vi "BindCluster.vi"(8 "error in (no error)":errorcluster, 9 "Controls[]":refnum<vi>[](array[refnum]), 10 "Cols":T2[](array[typedef])=[{"Include"=TRUE, "Name"="Position", "SQLite3 type"=enum."SQLITE_FLOAT"}, {"Include"=TRUE, "Name"="Event Type", "SQLite3 type"=enum."SQLITE_INTEGER"}, {"Include"=TRUE, "Name"="Area", "SQLite3 type"=enum."SQLITE_INTEGER"}, {"Include"=TRUE, "Name"="Channels", "SQLite3 type"=enum."SQLITE_INTEGER"}, {"Include"=TRUE, "Name"="Start position", "SQLite3 type"=enum."SQLITE_INTEGER"}, {"Include"=TRUE, "Name"="End  position", "SQLite3 type"=enum."SQLITE_INTEGER"}, {"Include"=TRUE, "Name"="Name", "SQLite3 type"=enum."SQLITE3_TEXT"}, {"Include"=TRUE, "Name"="Offset", "SQLite3 type"=enum."SQLITE_INTEGER"}, {"Include"=TRUE, "Name"="Length", "SQLite3 type"=enum."SQLITE_INTEGER"}, {"Include"=TRUE, "Name"="Action marker", "SQLite3 type"=enum."SQLITE3_TEXT"}, {"Include"=TRUE, "Name"="Event", "SQLite3 type"=enum."SQLITE_INTEGER"}, {"Include"=TRUE, "Name"="# Defects", "SQLite3 type"=enum."SQLITE_INTEGER"}, {"Include"=TRUE, "Name"="jpg Image", "SQLite3 type"=enum."SQLITE3_TEXT"}, {"Include"=TRUE, "Name"="chan maxs", "SQLite3 type"=enum."SQLITE_INTEGER"}, {"Include"=TRUE, "Name"="chan mins", "SQLite3 type"=enum."SQLITE_INTEGER"}, {"Include"=TRUE, "Name"="TimeStamp", "SQLite3 type"=enum."SQLITE_INTEGER"}, {"Include"=TRUE, "Name"="Readings", "SQLite3 type"=enum."SQLITE3_TEXT"}, {"Include"=TRUE, "Name"="ID", "SQLite3 type"=enum."SQLITE_INTEGER"}, {"Include"=TRUE, "Name"="New", "SQLite3 type"=enum."SQLITE_INTEGER"}, {"Include"=TRUE, "Name"="Hires Track", "SQLite3 type"=enum."SQLITE_INTEGER"}, {"Include"=FALSE, "Name"="2D overlay", "SQLite3 type"=enum."SQLITE_INTEGER"}, {"Include"=TRUE, "Name"="update", "SQLite3 type"=enum."SQLITE_INTEGER"}, {"Include"=TRUE, "Name"="Field #", "SQLite3 type"=enum."SQLITE_INTEGER"}, {"Include"=TRUE, "Name"="Events Class", "SQLite3 type"=enum."SQLITE_INTEGER"}, {"Include"=TRUE, "Name"="Sync", "SQLite3 type"=enum."SQLITE_INTEGER"}, {"Include"=TRUE, "Name"="Insert Offset", "SQLite3 type"=enum."SQLITE_INTEGER"}, {"Include"=TRUE, "Name"="Next trend", "SQLite3 type"=enum."SQLITE_INTEGER"}, {"Include"=TRUE, "Name"="Speed", "SQLite3 type"=enum."SQLITE_INTEGER"}], 11 "SQL Statement in":refnum<class "SQL Statement.lvclass">) -> (0 "error out":errorcluster, 2 "Array":string[](array[string]), 3 "SQL Statement out":refnum<class "SQL Statement.lvclass">, 5 "Time":u32)   [LabVIEW 2017, in "Copy of Beltwatch SQLite.lvlib"]
uses:
  Beltwatch/BeltWatch 4-2-2-5/Database/Copy of Beltwatch SQLite.lvlib
  <vilib>/drjdpowell/SQLite Library/SQL Statement/SQL Statement.lvclass
  Common64/Database/SQ Lite/SQ Lite Cluster Action.ctl
  <vilib>/Utility/Data Type/Type Definitions/Data Type.ctl
  <vilib>/drjdpowell/SQLite Library/SQL Statement/SQL Statement.lvclass/SQL Statement.ctl
  <vilib>/drjdpowell/SQLite Library/SQL Statement/Bind Integer.vi
  <vilib>/drjdpowell/SQLite Library/SQL Statement/Bind Blob.vi
  <vilib>/drjdpowell/SQLite Library/SQL Statement/Bind Null.vi
  <vilib>/drjdpowell/SQLite Library/SQL Statement/Bind Real.vi
  <vilib>/drjdpowell/SQLite Library/SQL Statement/Bind Text.vi
  <vilib>/drjdpowell/SQLite Library/SQL Statement/Error Message.vi
  <vilib>/Utility/Data Type/NI_Data Type.lvlib
panel:
  out "Type":T1
  out "Name":string
  out "Value":variant
  out "?":string
  out "Waveform Chart":u32(graph)
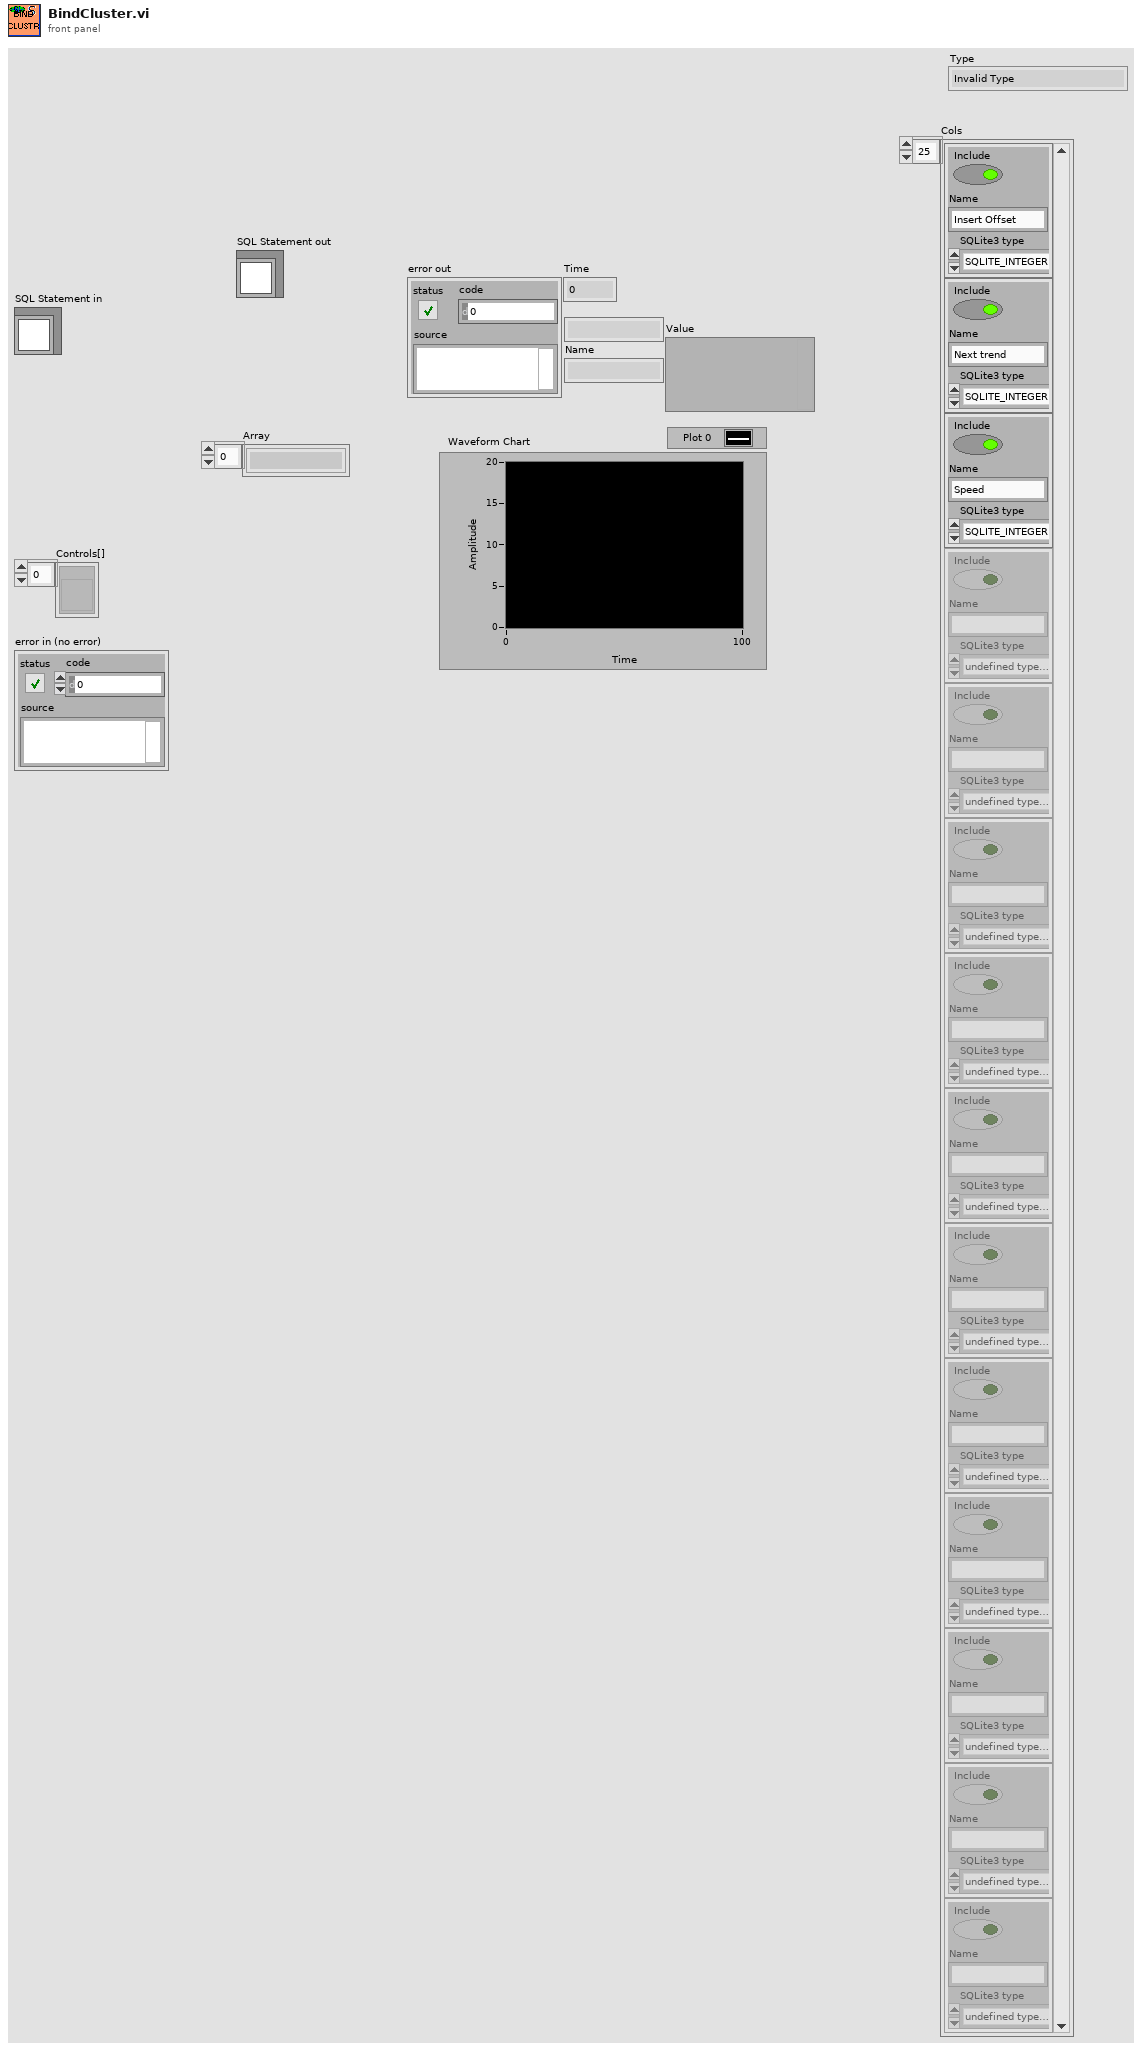
[diagram p1: front panel]
types:
  T1 = typedef "NI_Data Type.lvlib/Data Type.ctl" = enum8{"Invalid Type", "Void", "I8", "I16", "I32", "I64", "U8", "U16", "U32", "U64", "Single Float", "Double Float", "Extended Float", "Single Complex", "Double Complex", "Extended Complex", "Enum U8", "Enum U16", "Enum U32", "Enum U64", "Single Float With Unit", "Double Float With Unit", "Extended Float With Unit", "Single Complex with Unit", "Double Complex with Unit", "Extended Complex with Unit", "Boolean", "String", "Path", "Picture", "Tag", "Array", "Cluster", "Variant", "LV Variant", "Waveform", "Timestamp", "Digital Waveform", "Digital Data", "ExpressData", "Refnum", "External Data", "VI", "Poly VI", "LabVIEW Class Instance", "Fixed Point"}
  T2 = typedef "Copy of Beltwatch SQLite.lvlib/SQ Lite Cluster Action.ctl" = cluster{"Include":bool, "Name":string, "SQLite3 type":enum32{"undefined type (0)", "SQLITE_INTEGER", "SQLITE_FLOAT", "SQLITE3_TEXT", "SQLITE_BLOB", "SQLITE_NULL", "undefined type", "FloatArray"}}
  T3 = enum32{"undefined type (0)", "SQLITE_INTEGER", "SQLITE_FLOAT", "SQLITE3_TEXT", "SQLITE_BLOB", "SQLITE_NULL", "undefined type", "FloatArray"}
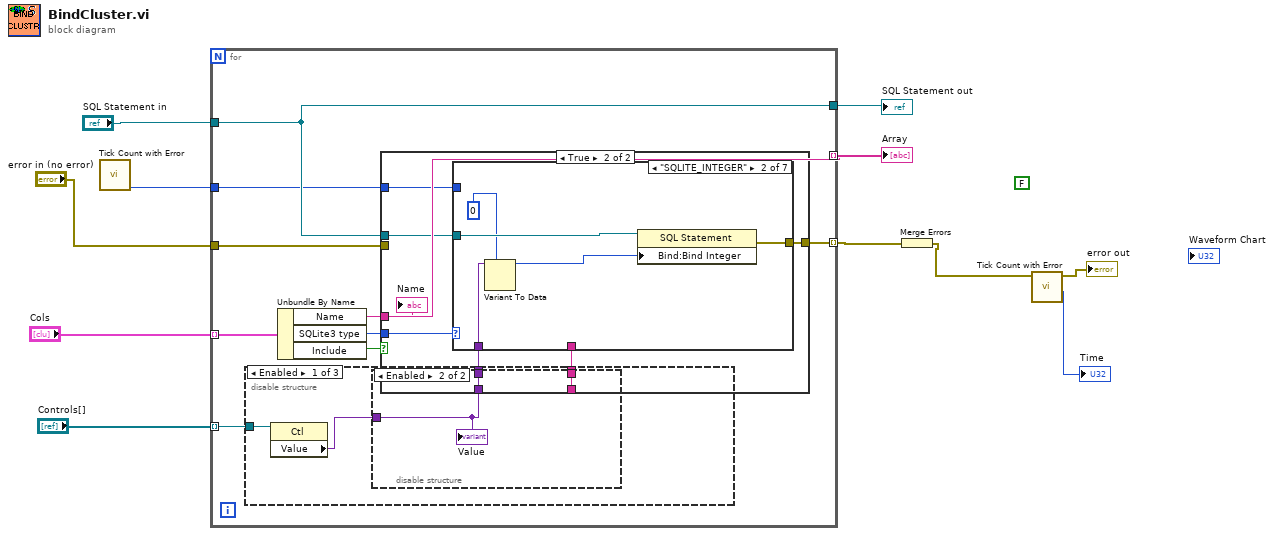
[diagram p0: block diagram]
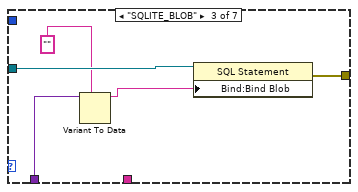
[diagram p4: hidden frame]
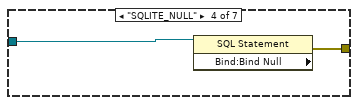
[diagram p5: hidden frame]
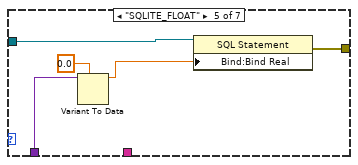
[diagram p6: hidden frame]
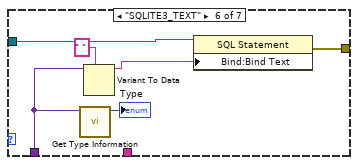
[diagram p7: hidden frame]
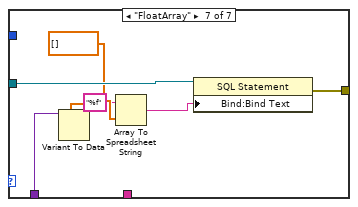
[diagram p8: hidden frame]
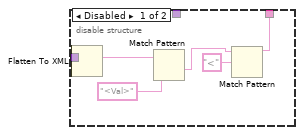
[diagram p9: hidden frame]
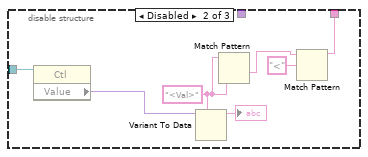
[diagram p10: hidden frame]
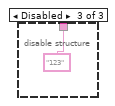
[diagram p11: hidden frame]
diagram:
  (unwired) FALSE ("UsePrevious")
  n1 = call "Tick Count with Error.vi"() -> ("millisecond timer value"=w5:u32)  [unwired: 9 in, 2 out]
  n2 = for {
    tunnel: "Cols" -> [w22] mode=indexing
    tunnel: "Controls[]" -> [w21] mode=indexing
    tunnel: [w19] -> w8 mode=indexing
    tunnel: w5 -> [w16]
    tunnel: "SQL Statement in" -> [w17]
    tunnel: [w17] -> w11
    tunnel: [w15] -> w6 mode=indexing
    tunnel: "error in (no error)" -> [w12]
    n3 = disable-structure shown="Enabled" {
      disable-tunnel: w21 -> [w62 w74 _]
      disable-tunnel: [w63 w75 "123" ("regular expression")] -> w18
      disable-tunnel: [w60 _ _] -> w14
      frame Enabled {
        n4 = property class="Ctl"(reference=w62) -> ("Value"=w61:variant)  [unwired: 1 in, 2 out]
        n5 = disable-structure shown="Enabled" {
          disable-tunnel: [w65 _] -> w63
          disable-tunnel: w61 -> [w64 w70]
          disable-tunnel: [_ w70] -> w60
          frame Disabled {
            n6 = Flatten To XML(anything=w64) -> (xml string=w69:string)
            n7 = Match Pattern(string=w69, regular expression="<Val>") -> (after substring=w67:string)  [unwired: 1 in, 3 out]
            n8 = Match Pattern(string=w67, regular expression="<") -> (before substring=w65:string)  [unwired: 1 in, 3 out]
          }
          frame Enabled {
            "Value" <- w70
          }
        }
      }
      frame Disabled {
        w71 = "<Val>" ("regular expression")
        n9 = property class="Ctl"(reference=w74) -> ("Value"=w73:variant)  [unwired: 1 in, 2 out]
        n10 = Variant To Data(type=w71, Variant=w73) -> (data=→"?":string)  [unwired: 1 in, 1 out]
        n11 = Match Pattern(string=w71, regular expression=w71) -> (after substring=w77:string)  [unwired: 1 in, 3 out]
        n12 = Match Pattern(string=w77, regular expression="<") -> (before substring=w75:string)  [unwired: 1 in, 3 out]
      }
      frame Disabled {
      }
    }
    n13 = Unbundle By Name(w22) -> ("Name"=w19:string, "SQLite3 type"=w20:T3, "Include"=w13:bool)
    n14 = case shown="True" w13 {
      tunnel: w20 -> [_ w30]
      tunnel: w19 -> [_ w29]
      tunnel: w18 -> [_ w28]
      tunnel: w17 -> [_ w27]
      tunnel: w16 -> [_ w26]
      tunnel: [w23 w25] -> w15
      tunnel: w14 -> [_ w24]
      tunnel: w12 -> [w23 _]
      frame False {
      }
      frame True {
        n15 = case shown="\"SQLITE_INTEGER\"" w30 {
          tunnel: w27 -> [_ w35 w40 w42 w47 w53 w59]
          tunnel: w28 -> [_ _ _ _ _ _ _]
          tunnel: w26 -> [_ _ _ _ _ _ _]
          tunnel: [_ w34 w39 w41 w46 w52 w58] -> w25
          tunnel: w24 -> [_ w33 w38 _ w43 w49 w57]
          frame "undefined type (0)", Default {
          }
          frame "SQLITE_INTEGER" {
            n16 = Variant To Data(type=0, Variant=w33) -> (data=w31:i32)  [unwired: 1 in, 1 out]
            n17 = property class="SQL Statement"(reference=w35, "Bind:Bind Integer"=w31) -> (error out=w34:errorcluster)  [unwired: 1 in, 1 out]
          }
          frame "SQLITE_BLOB" {
            n18 = Variant To Data(type="", Variant=w38) -> (data=w36:string)  [unwired: 1 in, 1 out]
            n19 = property class="SQL Statement"(reference=w40, "Bind:Bind Blob"=w36) -> (error out=w39:errorcluster)  [unwired: 1 in, 1 out]
          }
          frame "SQLITE_NULL" {
            n20 = property class="SQL Statement" props=["Bind:Bind Null"](reference=w42) -> (error out=w41:errorcluster)  [unwired: 1 in, 2 out]
          }
          frame "SQLITE_FLOAT" {
            n21 = Variant To Data(type=0.0, Variant=w43) -> (data=w44:dbl)  [unwired: 1 in, 1 out]
            n22 = property class="SQL Statement"(reference=w47, "Bind:Bind Real"=w44) -> (error out=w46:errorcluster)  [unwired: 1 in, 1 out]
          }
          frame "SQLITE3_TEXT" {
            n23 = call <vilib>:"Get Type Information.vi"("Variant"=w49) -> ("Type"=→"Type":T1)  [unwired: 6 in, 4 out]
            n24 = Variant To Data(type=" ", Variant=w49) -> (data=w50:string)  [unwired: 1 in, 1 out]
            n25 = property class="SQL Statement"(reference=w53, "Bind:Bind Text"=w50) -> (error out=w52:errorcluster)  [unwired: 1 in, 1 out]
          }
          frame "FloatArray" {
            w56 = dbl[] []
            n26 = Variant To Data(type=w56, Variant=w57) -> ()  [unwired: 1 in, 2 out]
            n27 = Array To Spreadsheet String(array=w56, 3:"%f" ("format string")) -> (spreadsheet string=w55:string)  [unwired: 1 in]
            n28 = property class="SQL Statement"(reference=w59, "Bind:Bind Text"=w55) -> (error out=w58:errorcluster)  [unwired: 1 in, 1 out]
          }
        }
        "Name" <- w29
      }
    }
  }
  "SQL Statement out" <- w11
  "Array" <- w8
  n29 = Merge Errors(w6) -> (w4:errorcluster)
  n30 = call "Tick Count with Error.vi"("error in (no error)"=w4) -> ("Time"=→"Time":u32, "error out"=→"error out":errorcluster)  [unwired: 8 in, 1 out]
